vi "F Random.vi"(6 "seed":i32=-1, 7 "reset":bool, 9 "k2":i32=1, 10 "k1":i32=1, 11 "samples":i32=128) -> (0 "error":i32, 3 "f random numbers":dbl[](array[numeric]))   [LabVIEW 2020, in "NI_Gmath.lvlib"]
doc: "Generates random values from a variate X, where X describes the selected distribution type. You must manually select the polymorphic instance to use."
uses:
  NI_Gmath.lvlib
panel:
  # "F Random"
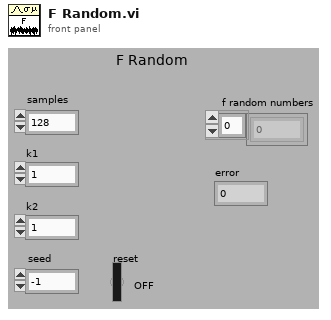
[diagram p1: front panel]
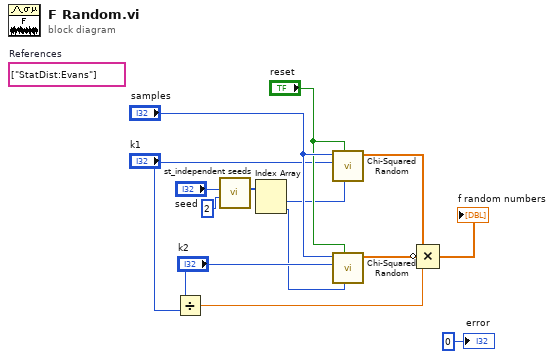
[diagram p0: block diagram]
diagram:
  (unwired) string[] ["StatDist:Evans"]  # References
  n1 = Divide(x="k2", y="k1") -> (x/y=w2:dbl)
  n2 = call "st_independent seeds.vi"("number of seeds"=2, "seed"="seed") -> ("independent seeds"=w4:i32[])  [unwired: 9 in]
  n3 = Index Array(array=w4) -> (element #1=w3:i32, element #2=w1:i32)  [unwired: 2 in]
  n4 = call "Chi-Squared Random.vi"("seed"=w3, "reset"="reset", "k"="k1", "samples"="samples") -> ("chi-squared random data"=w11:dbl[])  [unwired: 6 in, 1 out]
  n5 = call "Chi-Squared Random.vi"("seed"=w1, "reset"="reset", "k"="k2", "samples"="samples") -> ("chi-squared random data"=w10:dbl[])  [unwired: 6 in, 1 out]
  n6 = Compound Arithmetic op=MULTIPLY(w11, invert w10, w2) -> (→"f random numbers":dbl[])
  "error" <- 0 ("error")
